vi "Convert String to Time Stamp.vi"(7 "default value of time stamp":timestamp, 11 "string":string) -> (3 "time stamp out":timestamp format="%<%Y-%m-%dT%H:%M:%S%8u\nTime zone offset %z>T")   [LabVIEW 2020, in "infolib.lvlib"]
doc: "converts string to time stamp according ISO"
uses:
  infolib.lvlib
  <vilib>/Utility/miscctls.llb/LVDateTimeRec.ctl
  <vilib>/regexp/Match Regular Expression.xnode
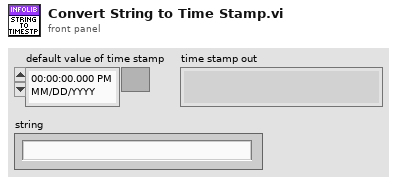
[diagram p1: front panel]
types:
  T1 = typedef "LVDateTimeRec.ctl" = cluster{"fractional second":dbl, "second":i32, "minute":i32, "hour":i32, "day of month":i32, "month":i32, "year":i32, "day of week":i32, "day of year":i32, "DST":i32}
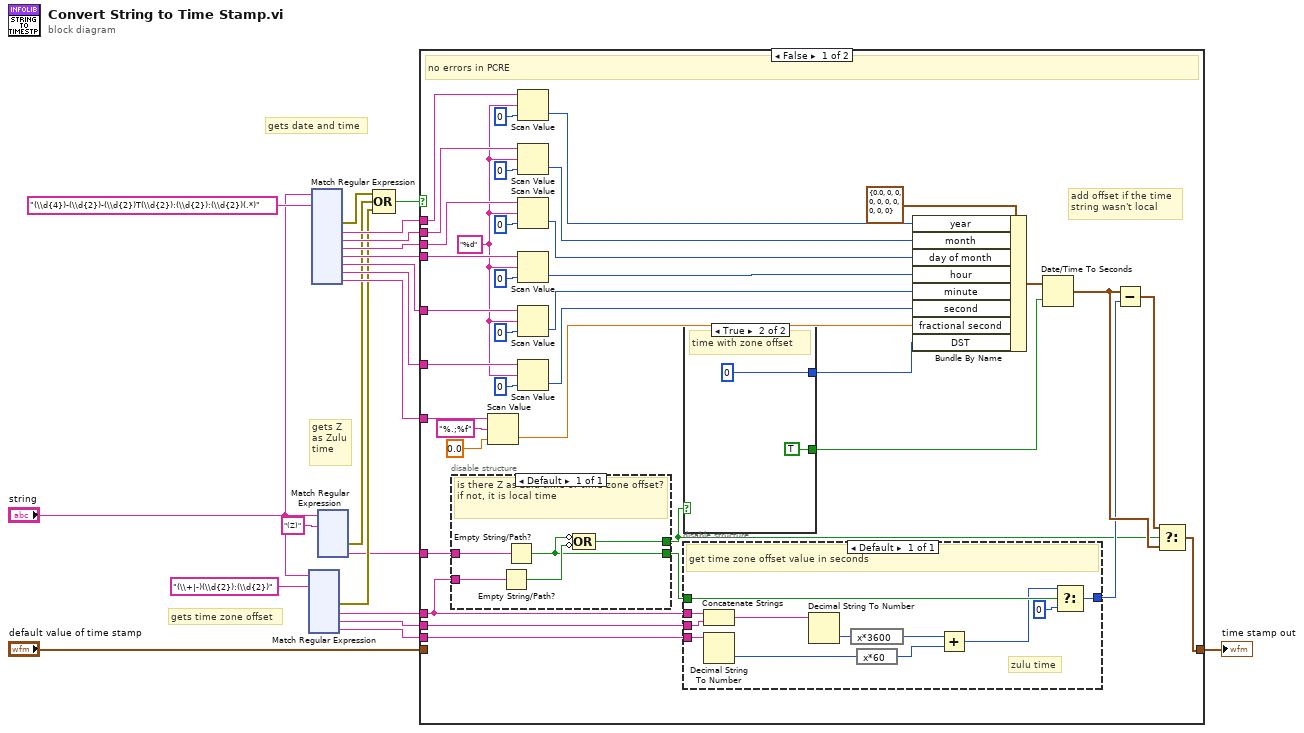
[diagram p0: block diagram]
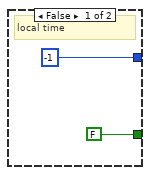
[diagram p2: hidden frame]
diagram:
  # "gets time zone offset"
  # "gets Z\nas Zulu\ntime"
  # "gets date and time"
  n1 = xnode "Match Regular Expression"("input string"="string", "regular expression"="(\\+|-)(\\d{2}):(\\d{2})") -> ("error out"=w6:errorcluster, "submatch 1"=w3:string, "submatch 2"=w2:string, "submatch 3"=w1:string)  [unwired: 4 in, 4 out]
  n2 = xnode "Match Regular Expression"("input string"="string", "regular expression"="(\\d{4})-(\\d{2})-(\\d{2})T(\\d{2}):(\\d{2}):(\\d{2})(.*)") -> ("error out"=w8:errorcluster, "submatch 1"=w13:string, "submatch 2"=w15:string, "submatch 3"=w16:string, "submatch 4"=w17:string, "submatch 5"=w18:string, "submatch 6"=w19:string, "submatch 7"=w20:string)  [unwired: 4 in, 4 out]
  n3 = xnode "Match Regular Expression"("input string"="string", "regular expression"="(Z)") -> ("error out"=w7:errorcluster, "submatch 1"=w4:string)  [unwired: 4 in, 4 out]
  n4 = Compound Arithmetic op=OR(w8, w7, w6) -> (w5:bool)
  n5 = case shown="False" w5 {
    tunnel: w13 -> [w58 _]
    tunnel: [w30 w80] -> w14
    tunnel: w15 -> [w51 _]
    tunnel: w16 -> [w49 _]
    tunnel: w17 -> [w46 _]
    tunnel: w18 -> [w43 _]
    tunnel: w19 -> [w40 _]
    tunnel: w20 -> [w37 _]
    tunnel: "default value of time stamp" -> [_ w80]
    tunnel: w4 -> [w28 _]
    tunnel: w3 -> [w27 _]
    tunnel: w2 -> [w26 _]
    tunnel: w1 -> [w25 _]
    frame False {
      w35 = "%d" ("format string")
      # "add offset if the time\nstring wasn't local"
      # "no errors in PCRE"
      n6 = disable-structure shown="Default" {
        disable-tunnel: [w62] -> w29
        disable-tunnel: w28 -> [w61]
        disable-tunnel: w27 -> [w60]
        disable-tunnel: [w59] -> w23
        frame Enabled {
          # "is there Z as zulu time or time zone offset? if not, it is local time"
          n7 = Empty String/Path?(string/path=w60) -> (empty?=w63:bool)
          n8 = Empty String/Path?(string/path=w61) -> (empty?=w62:bool)
          n9 = Compound Arithmetic op=OR(invert w62, invert w63) -> (w59:bool)
        }
      }
      n10 = Scan Value(string=w37, format string="%.;%f", default (0 dbl)=0.0) -> (value=w36:dbl)  [unwired: 1 out]
      n11 = Scan Value(string=w58, format string=w35, default (0 dbl)=0) -> (value=w53:i32)  [unwired: 1 out]
      n12 = Scan Value(string=w51, format string=w35, default (0 dbl)=0) -> (value=w52:i32)  [unwired: 1 out]
      n13 = Scan Value(string=w49, format string=w35, default (0 dbl)=0) -> (value=w48:i32)  [unwired: 1 out]
      n14 = Scan Value(string=w46, format string=w35, default (0 dbl)=0) -> (value=w45:i32)  [unwired: 1 out]
      n15 = Scan Value(string=w43, format string=w35, default (0 dbl)=0) -> (value=w42:i32)  [unwired: 1 out]
      n16 = Scan Value(string=w40, format string=w35, default (0 dbl)=0) -> (value=w39:i32)  [unwired: 1 out]
      n17 = case shown="True" w23 {
        tunnel: [-1 ("DST") 0 ("DST")] -> w33
        tunnel: [FALSE ("is UTC (F)") TRUE ("is UTC (F)")] -> w22
        frame False {
          # "local time"
        }
        frame True {
          # "time with zone offset"
        }
      }
      n18 = disable-structure shown="Default" {
        disable-tunnel: w29 -> [w75]
        disable-tunnel: w27 -> [w67]
        disable-tunnel: w26 -> [w66]
        disable-tunnel: w25 -> [w65]
        disable-tunnel: [w64] -> w24
        frame Enabled {
          # "zulu time"
          # "get time zone offset value in seconds"
          n19 = Concatenate Strings(w67, w66) -> (w68:string)
          n20 = Decimal String To Number(string=w65) -> (number=w70:i32)  [unwired: 2 in, 1 out]
          n21 = Decimal String To Number(string=w68) -> (number=w69:i32)  [unwired: 2 in, 1 out]
          n22 = expression code="x*3600"(w69) -> (w71:i32)
          n23 = expression code="x*60"(w70) -> (w72:i32)
          n24 = Add(x=w71, y=w72) -> (x+y=w73:i32)
          n25 = Select(t=w73, s=w75, f=0) -> (s? t:f=w64:i32)
        }
      }
      n26 = Bundle By Name(cluster=T1 {"fractional second"=0.0, "second"=0, "minute"=0, "hour"=0, "day of month"=0, "month"=0, "year"=0, "day of week"=0, "day of year"=0, "DST"=0} ("date time rec"), "year"=w53, "month"=w52, "day of month"=w48, "hour"=w45, "minute"=w42, "second"=w39, "fractional second"=w36, "DST"=w33) -> (w54:T1)
      n27 = Date/Time To Seconds(1:w22, 2:w54) -> (0:w31:timestamp)
      n28 = Subtract(x=w31, y=w24) -> (x-y=w32:timestamp)
      n29 = Select(t=w32, s=w23, f=w31) -> (s? t:f=w30:timestamp)
    }
    frame True {
    }
  }
  "time stamp out" <- w14
